vi "ASCII Actor.vi"(11 "VISA resource name":refnum<visa-resource-name>) -> (0 "error out":errorcluster)   [LabVIEW 2019, in "ASCII Actor.lvlib"]
uses:
  ASCII Actor.lvlib
  <vilib>/Instr/_visa.llb/VISA Configure Serial Port (Instr).vi
  Queue Task.ctl
  Actor Task.ctl
  Actor Command.ctl
panel:
  out "read buffer":string
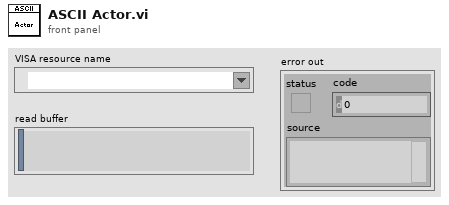
[diagram p1: front panel]
types:
  T1 = typedef "ASCII Actor.lvlib/Actor Command.ctl" = cluster{"Task":T2, "Data":string, "Response Queue":refnum<queue>}
  T2 = typedef "ASCII Actor.lvlib/Actor Task.ctl" = enum8{"Write", "Get Data", "Stop"}
  T3 = typedef "ASCII Actor.lvlib/Queue Task.ctl" = enum8{"Get Reference", "Send", "Close"}
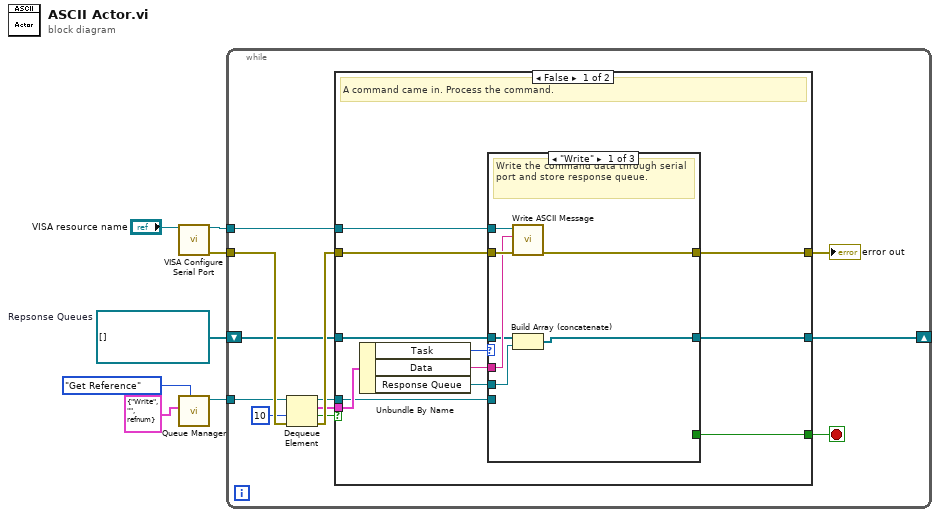
[diagram p0: block diagram]
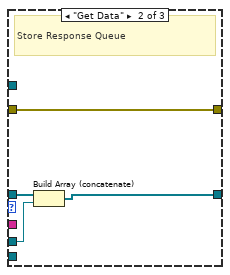
[diagram p2: hidden frame]
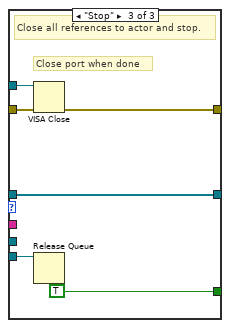
[diagram p3: hidden frame]
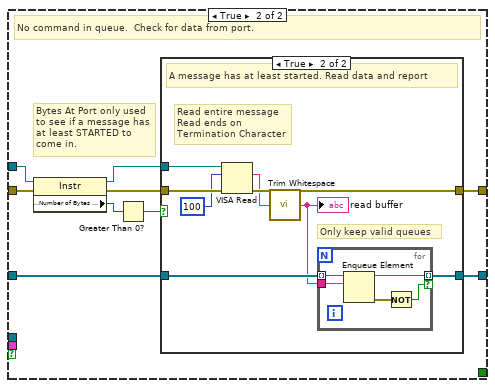
[diagram p4: hidden frame]
diagram:
  w2 = refnum<queue>[] []  # Repsonse Queues
  n1 = call-poly "VISA Configure Serial Port"("VISA resource name"="VISA resource name") -> ("VISA resource name out"=w5:refnum<visa-resource-name>, "error out"=w7:errorcluster)  [unwired: 13 in]
  n2 = call "Queue Manager.vi"("Task"=Queue_Task."Get Reference", "Command"=T1 {"Task"=enum."Write", "Data"="", "Response Queue"=refnum}) -> ("Queue"=w4:refnum<queue>)  [unwired: 8 in, 1 out]
  n3 = while {
    tunnel: w7 -> [w18]
    tunnel: w5 -> [w16]
    tunnel: w4 -> [w15]
    shift-right: [w10] -> _
    shift-left: w2 -> [w11]
    stop <- w8 stop-if-true
    n4 = Dequeue Element(queue=w15, timeout in ms (-1)=10, error in (no error)=w18) -> (queue out=w9:refnum<queue>, element=w12:T1, timed out?=w13:bool, error out=w19:errorcluster)
    n5 = case shown="False" w13 {
      tunnel: [w29 w55] -> w17
      tunnel: w16 -> [w24 w53]
      tunnel: w19 -> [w30 w54]
      tunnel: w12 -> [w28 _]
      tunnel: w11 -> [w23 w49]
      tunnel: [w22 w48] -> w10
      tunnel: w9 -> [w21 _]
      tunnel: [w20 _] -> w8
      frame False {
        # "A command came in. Process the command."
        n6 = Unbundle By Name(w28) -> ("Task"=w25:T2, "Data"=w26:string, "Response Queue"=w27:refnum<queue>)
        n7 = case shown="\"Write\"" w25 {
          tunnel: w27 -> [w32 w38 _]
          tunnel: w26 -> [w34 _ _]
          tunnel: w24 -> [w35 _ w45]
          tunnel: w23 -> [w33 w40 w43]
          tunnel: [w31 w39 w43] -> w22
          tunnel: w30 -> [w37 w41 w47]
          tunnel: [w36 w41 w46] -> w29
          tunnel: w21 -> [_ _ w44]
          tunnel: [_ _ TRUE] -> w20
          frame "Write" {
            # "Write the command data through serial port and store response queue."
            n8 = call "Write ASCII Message.vi"("error in"=w37, "Message"=w34, "VISA resource in"=w35) -> ("error out"=w36:errorcluster)  [unwired: 7 in, 1 out]
            n9 = Build Array (concatenate)(w33, w32) -> (w31:refnum<queue>[])
          }
          frame "Get Data" {
            # "Store Response Queue"
            n10 = Build Array (concatenate)(w40, w38) -> (w39:refnum<queue>[])
          }
          frame "Stop" {
            # "Close port when done"
            # "Close all references to actor and stop."
            n11 = VISA Close(VISA resource name=w45, error in (no error)=w47) -> (error out=w46:errorcluster)
            n12 = Release Queue(queue=w44) -> ()  [unwired: 2 in, 3 out]
          }
        }
      }
      frame True {
        # "Bytes At Port only used\nto see if a message has\nat least STARTED to\ncome in."
        # "No command in queue.  Check for data from port."
        n13 = property class="Instr"(reference=w53, error in=w54) -> (reference out=w50:refnum<visa-resource-name>, error out=w56:errorcluster, "Serial Settings:Number of Bytes at Serial Port"=w52:u32)
        n14 = Greater Than 0?(x=w52) -> (x > 0?=w51:bool)
        n15 = case shown="True" w51 {
          tunnel: w56 -> [w58 w66]
          tunnel: w50 -> [_ w64]
          tunnel: [w58 w65] -> w55
          tunnel: w49 -> [w57 w61]
          tunnel: [w57 w59] -> w48
          frame False {
            # "No message. Go back to waiting for a command."
          }
          frame True {
            # "Only keep valid queues"
            # "Read entire message\nRead ends on\nTermination Character"
            # "A message has at least started. Read data and report"
            n16 = VISA Read(VISA resource name=w64, byte count=u32 100, error in (no error)=w66) -> (read buffer=w62:string, error out=w65:errorcluster)  [unwired: 2 out]
            n17 = call <vilib>:"Trim Whitespace.vi"("string"=w62) -> ("trimmed string"=w60:string)  [unwired: 1 in]
            "read buffer" <- w60
            n18 = for {
              tunnel: w61 -> [w70] mode=indexing
              tunnel: w60 -> [w69]
              tunnel: [w68] -> w59 mode=indexing if=w67
              n19 = Enqueue Element(queue=w70, element=w69) -> (queue out=w68:refnum<queue>, error out=w71:errorcluster)  [unwired: 2 in, 1 out]
              n20 = Not(x=w71) -> (.not. x?=w67:bool)
            }
          }
        }
      }
    }
    "error out" <- w17
  }
